vi "Logo.vi"() -> ()   [LabVIEW 2015]
uses:
  USER32.DLL
panel:
  in  "string1":string="CHEN"
  in  "string2":string="勤眾興業"
  in  "Color Box":u32(colorbox)=46079
  in  "CHEN":bool
  out "LOGO":T1
  in  "CHEN 2":bool
  in  "Color Box 2":u32(colorbox)=56466
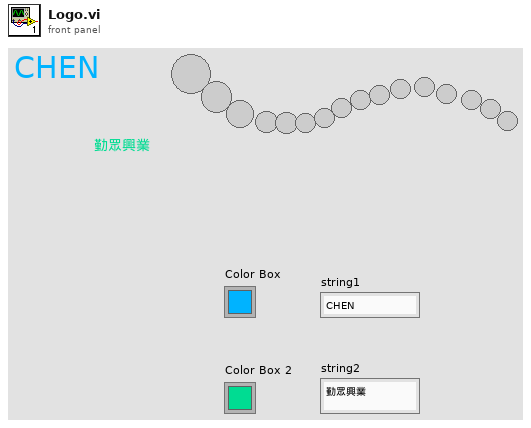
[diagram p1: front panel]
types:
  T1 = cluster{"Round Color Box 72":u32, "Round Color Box 73":u32, "Round Color Box 74":u32, "Round Color Box 75":u32, "Round Color Box 76":u32, "Round Color Box 77":u32, "Round Color Box 78":u32, "Round Color Box 79":u32, "Round Color Box 80":u32, "Round Color Box 65":u32, "Round Color Box 66":u32, "Round Color Box 67":u32, "Round Color Box 68":u32, "Round Color Box 69":u32, "Round Color Box 70":u32, "Round Color Box 71":u32}
  T2 = cluster{"[0]":u32, "[1]":u32, "[2]":u32, "[3]":u32, "[4]":u32, "[5]":u32, "[6]":u32, "[7]":u32, "[8]":u32, "[9]":u32, "[10]":u32, "[11]":u32, "[12]":u32, "[13]":u32, "[14]":u32, "[15]":u32, "[16]":u32, "[17]":u32, "[18]":u32, "[19]":u32, "[20]":u32, "[21]":u32, "[22]":u32, "[23]":u32, "[24]":u32, "[25]":u32, "[26]":u32, "[27]":u32, "[28]":u32, "[29]":u32, "[30]":u32, "[31]":u32, "[32]":u32, "[33]":u32, "[34]":u32, "[35]":u32, "[36]":u32, "[37]":u32, "[38]":u32, "[39]":u32, "[40]":u32, "[41]":u32, "[42]":u32, "[43]":u32, "[44]":u32, "[45]":u32, "[46]":u32, "[47]":u32, "[48]":u32, "[49]":u32, "[50]":u32, "[51]":u32, "[52]":u32, "[53]":u32, "[54]":u32, "[55]":u32, "[56]":u32, "[57]":u32, "[58]":u32, "[59]":u32, "[60]":u32, "[61]":u32, "[62]":u32, "[63]":u32, "[64]":u32, "[65]":u32, "[66]":u32, "[67]":u32, "[68]":u32, "[69]":u32, "[70]":u32, "[71]":u32, "[72]":u32, "[73]":u32, "[74]":u32, "[75]":u32, "[76]":u32, "[77]":u32, "[78]":u32, "[79]":u32, "[80]":u32, "[81]":u32, "[82]":u32, "[83]":u32, "[84]":u32, "[85]":u32, "[86]":u32, "[87]":u32, "[88]":u32, "[89]":u32, "[90]":u32, "[91]":u32, "[92]":u32, "[93]":u32, "[94]":u32, "[95]":u32, "[96]":u32, "[97]":u32, "[98]":u32, "[99]":u32, "[100]":u32, "[101]":u32, "[102]":u32, "[103]":u32, "[104]":u32, "[105]":u32, "[106]":u32, "[107]":u32, "[108]":u32, "[109]":u32, "[110]":u32, "[111]":u32, "[112]":u32, "[113]":u32, "[114]":u32, "[115]":u32, "[116]":u32, "[117]":u32, "[118]":u32, "[119]":u32, "[120]":u32, "[121]":u32, "[122]":u32, "[123]":u32, "[124]":u32, "[125]":u32, "[126]":u32, "[127]":u32}
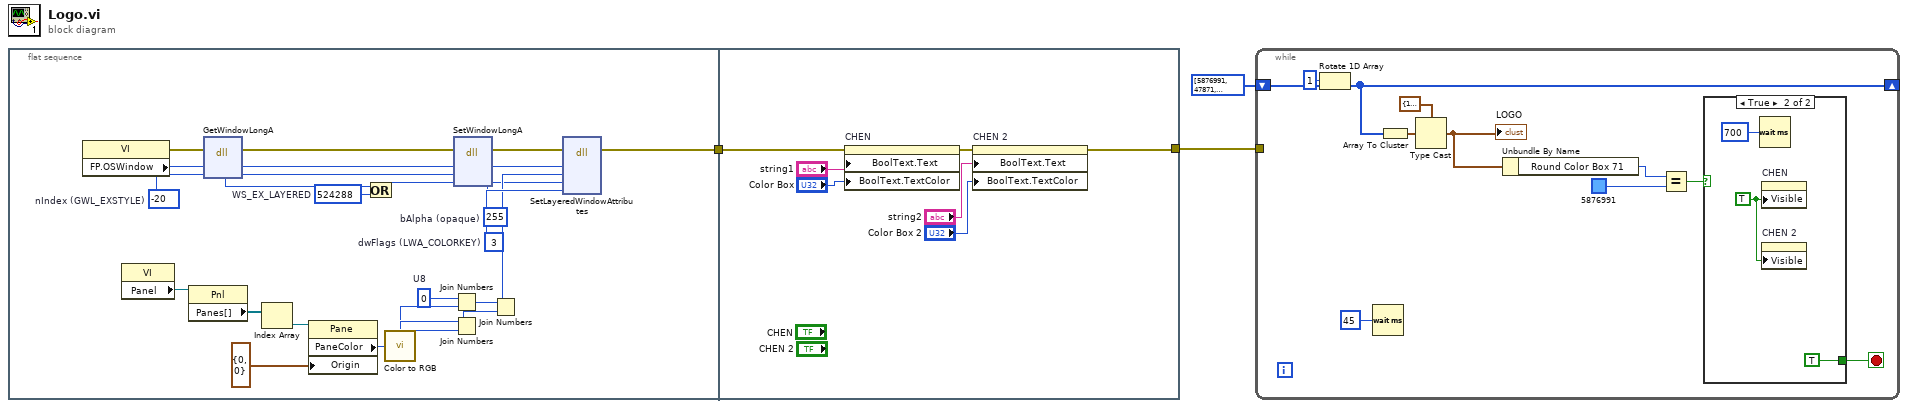
[diagram p0: block diagram]
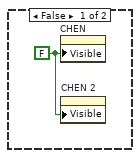
[diagram p2: hidden frame]
diagram:
  n1 = flat-sequence {
    tunnel: [w5] -> w2
    tunnel: w2 -> [w32]
    tunnel: [w30] -> w1
    frame #0 {
      w18 = 524288  # WS_EX_LAYERED
      w15 = -20  # nIndex (GWL_EXSTYLE)
      w21 = 255  # bAlpha (opaque)
      w22 = u8 0  # U8
      w26 = 3  # dwFlags (LWA_COLORKEY)
      n2 = property class="VI"() -> (error out=w13:errorcluster, "FP.OSWindow"=w17:i32)  [unwired: 2 in, 1 out]
      n3 = property class="VI"() -> ("Panel"=w29:refnum<vi>)  [unwired: 2 in, 2 out]
      n4 = property class="Pnl"(reference=w29) -> ("Panes[]"=w28:refnum<vi>[])  [unwired: 1 in, 2 out]
      n5 = dll-call lib="USER32.DLL" fn="GetWindowLongA" label="getWindowLong"(error in=w13, "handle"=w17, "nIndex"=w15) -> (error out=w12:errorcluster, w19:i32, "handle"=w16:i32, "nIndex"=w14:i32)  [unwired: 2 in, 1 out]
      n6 = Index Array(array=w28) -> (element=w27:refnum<vi>)  [unwired: 1 in]
      n7 = property class="Pane"(reference=w27, "Origin"=cluster{"right":i16, "bottom":i16} {"right"=0, "bottom"=0} ("Size")) -> ("PaneColor"=w9:u32)  [unwired: 1 in, 2 out]
      n8 = Or(x=w19, y=w18) -> (x .or. y?=w20:i32)
      n9 = call <vilib>:"Color to RGB.vi"("Color"=w9) -> ("R"=w8:u8, "G"=w7:u8, "B"=w6:u8)  [unwired: 1 out]
      n10 = Join Numbers(hi=w22, lo=w6) -> ((hi.lo)=w24:u16)
      n11 = Join Numbers(hi=w7, lo=w8) -> ((hi.lo)=w25:u16)
      n12 = dll-call lib="USER32.DLL" fn="SetWindowLongA" label="SetWindowLong"(error in=w12, "handle"=w16, "nIndex"=w14, "dwNewLong"=w20) -> (error out=w11:errorcluster, "handle"=w10:i32)  [unwired: 4 in, 2 out]
      n13 = Join Numbers(hi=w24, lo=w25) -> ((hi.lo)=w23:u32)
      n14 = dll-call lib="USER32.DLL" fn="SetLayeredWindowAttributes" label="SetLayerdWindowAttributs"(error in=w11, "handle"=w10, "crkey"=w23, "bAlpha"=w21, "dwFlags"=w26) -> (error out=w5:errorcluster)  [unwired: 6 in, 2 out]
    }
    frame #1 {
      n15 = property on="CHEN" class="Bool (strict)"(error in=w32, "BoolText.Text"="string1", "BoolText.TextColor"="Color Box") -> (error out=w31:errorcluster)  [unwired: 1 in, 1 out]
      n16 = property on="CHEN 2" class="Bool (strict)"(error in=w31, "BoolText.Text"="string2", "BoolText.TextColor"="Color Box 2") -> (error out=w30:errorcluster)  [unwired: 1 in, 1 out]
    }
  }
  n17 = while {
    shift-right: [w46] -> _
    shift-left: u32[] [5876991, 47871, 5887743, 10542847, 13629695, 15204345, 15204345, 15204345, 15204345, 15204345, 15204345, 15204345, 15204345, 15204345, 15204345, 15204345, 15204345, 15204345, 15204345] ("Array") -> [w47]
    tunnel: w1 -> [_]
    stop <- w37 stop-if-true
    n18 = Rotate 1D Array(1:w47, 2:1 ("n")) -> (0:w46:u32[])
    n19 = Wait (ms)(milliseconds to wait=u32 45) -> ()  [unwired: 1 out]
    n20 = Array To Cluster(array=w46) -> (cluster=w45:T2)
    n21 = Type Cast(type=T1 {"Round Color Box 72"=10542847, "Round Color Box 73"=5887743, "Round Color Box 74"=47871, "Round Color Box 75"=5876991, "Round Color Box 76"=15204345, "Round Color Box 77"=15204345, "Round Color Box 78"=15204345, "Round Color Box 79"=15204345, "Round Color Box 80"=15204345, "Round Color Box 65"=15204345, "Round Color Box 66"=15204345, "Round Color Box 67"=15204345, "Round Color Box 68"=15204345, "Round Color Box 69"=15204345, "Round Color Box 70"=15204345, "Round Color Box 71"=13629695} ("Cluster 11"), x=w45) -> (*(type *) &x=w42:T1)
    "LOGO" <- w42
    n22 = Unbundle By Name(w42) -> ("Round Color Box 71"=w41:u32)
    n23 = Equal?(x=w41, y=u32 5876991 ("Round Color Box")) -> (x = y?=w39:bool)
    n24 = case shown="True" w39 {
      tunnel: [_ TRUE ("stop 2")] -> w37
      frame False {
        w48 = FALSE ("Visible")
        n25 = property on="CHEN" class="Bool (strict)"("Visible"=w48) -> ()  [unwired: 2 in, 2 out]
        n26 = property on="CHEN 2" class="Bool (strict)"("Visible"=w48) -> ()  [unwired: 2 in, 2 out]
      }
      frame True {
        w50 = TRUE ("Visible")
        n27 = Wait (ms)(milliseconds to wait=u32 700) -> ()  [unwired: 1 out]
        n28 = property on="CHEN" class="Bool (strict)"("Visible"=w50) -> ()  [unwired: 2 in, 2 out]
        n29 = property on="CHEN 2" class="Bool (strict)"("Visible"=w50) -> ()  [unwired: 2 in, 2 out]
      }
    }
  }
